vi "Model - Init.vi"(8 "error in (no error)":errorcluster) -> (0 "error out":errorcluster, 3 "View Model":T1)   [LabVIEW 2017]
doc: "Initialize all components of View Model."
uses:
  Controls/View Model.ctl
  Controls/Shared Model.ctl
  Error Handler/Controls/Error Model.ctl
  Error Handler/Controls/Error Data.ctl
  Error Handler/Controls/Error Level.ctl
  Configuration/Controls/Config Model.ctl
  Configuration/Controls/Config Data Record.ctl
  Configuration/Controls/Config Command.ctl
  Controller/Controls/Control Model.ctl
  Controller/Controls/Elevator Location.ctl
  Controller/Controls/Elevator Status.ctl
  Controller/Controls/Control Event.ctl
  Controller/Controls/Control CMD.ctl
  Controller/Controls/Controller - Overhead.ctl
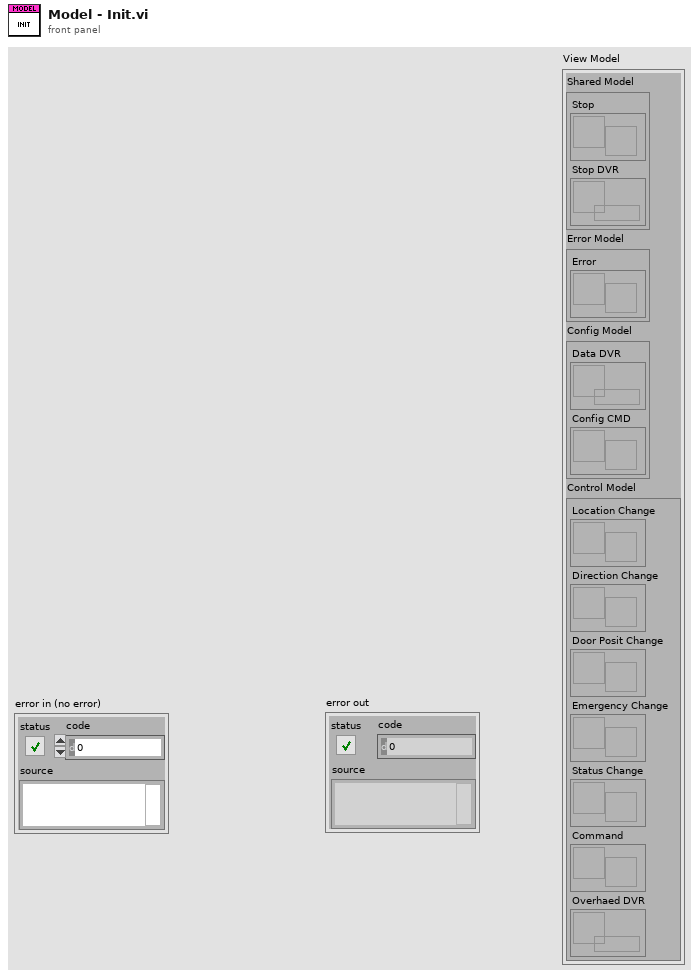
[diagram p1: front panel]
types:
  T1 = typedef "View Model.ctl" = cluster{"Shared Model":T2, "Error Model":T3, "Config Model":T4, "Control Model":T5}
  T2 = typedef "Shared Model.ctl" = cluster{"Stop":refnum<user-event>, "Stop DVR":refnum<data-value>}
  T3 = typedef "Error Model.ctl" = cluster{"Error":refnum<user-event>}
  T4 = typedef "Config Model.ctl" = cluster{"Data DVR":refnum<data-value>, "Config CMD":refnum<user-event>}
  T5 = typedef "Control Model.ctl" = cluster{"Location Change":refnum<user-event>, "Direction Change":refnum<user-event>, "Door Posit Change":refnum<user-event>, "Emergency Change":refnum<user-event>, "Status Change":refnum<user-event>, "Command":refnum<user-event>, "Overhaed DVR":refnum<data-value>}
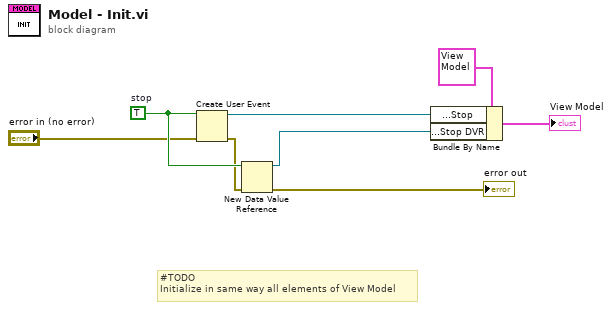
[diagram p0: block diagram]
diagram:
  w6 = TRUE  # stop
  # "#TODO\nInitialize in same way all elements of View Model"
  n1 = Create User Event(user event datatype=w6, error in="error in (no error)") -> (user event=w3:refnum<user-event>, error out=w4:errorcluster)
  n2 = New Data Value Reference(data value=w6, error in=w4) -> (data value reference=w2:refnum<data-value>, error out=→"error out":errorcluster)
  n3 = Bundle By Name(cluster=T1 {"Shared Model"={"Stop"=refnum, "Stop DVR"=refnum}, "Error Model"={"Error"=refnum}, "Config Model"={"Data DVR"=refnum, "Config CMD"=refnum}, "Control Model"={"Location Change"=refnum, "Direction Change"=refnum, "Door Posit Change"=refnum, "Emergency Change"=refnum, "Status Change"=refnum, "Command"=refnum, "Overhaed DVR"=refnum}} ("View Model"), "Shared Model.Stop"=w3, "Shared Model.Stop DVR"=w2) -> (→"View Model":T1)
